vi "LabVIEW RTE Debugging Viewer.vi"() -> ()   [LabVIEW 2015]
panel:
  in  "use default":bool=TRUE
  in  "Application to Debug":u16(ring)
  in  "autoRefresh":bool=TRUE
  in  "Refresh Button":bool
  in  "VIs Currently Loaded in Selected Application":i32(listbox)
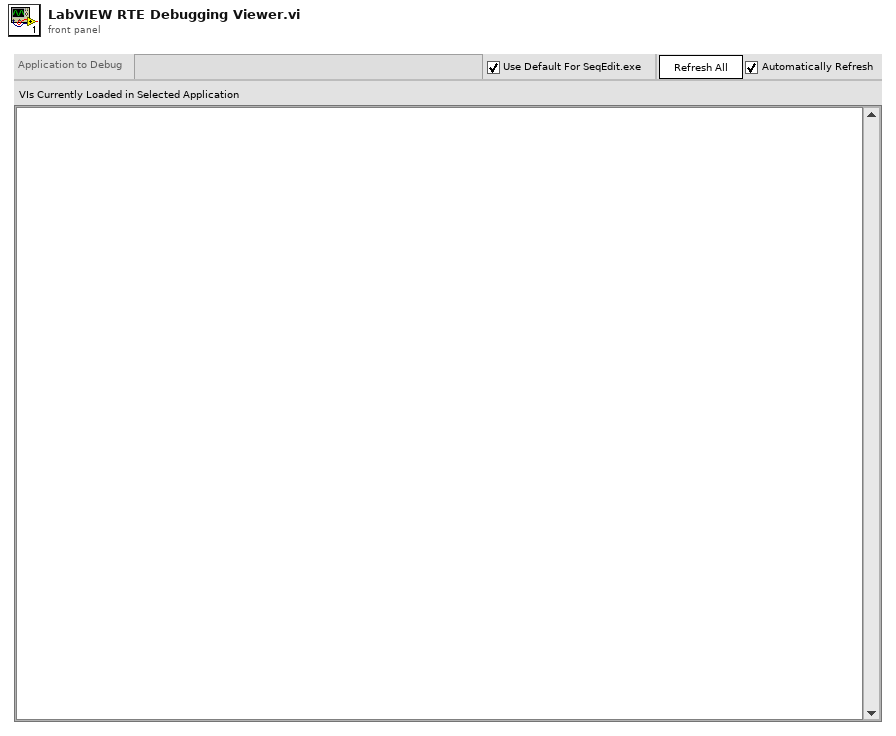
[diagram p1: front panel]
types:
  T1 = enum8{"Enabled", "Disabled", "Disabled and Grayed Out"}
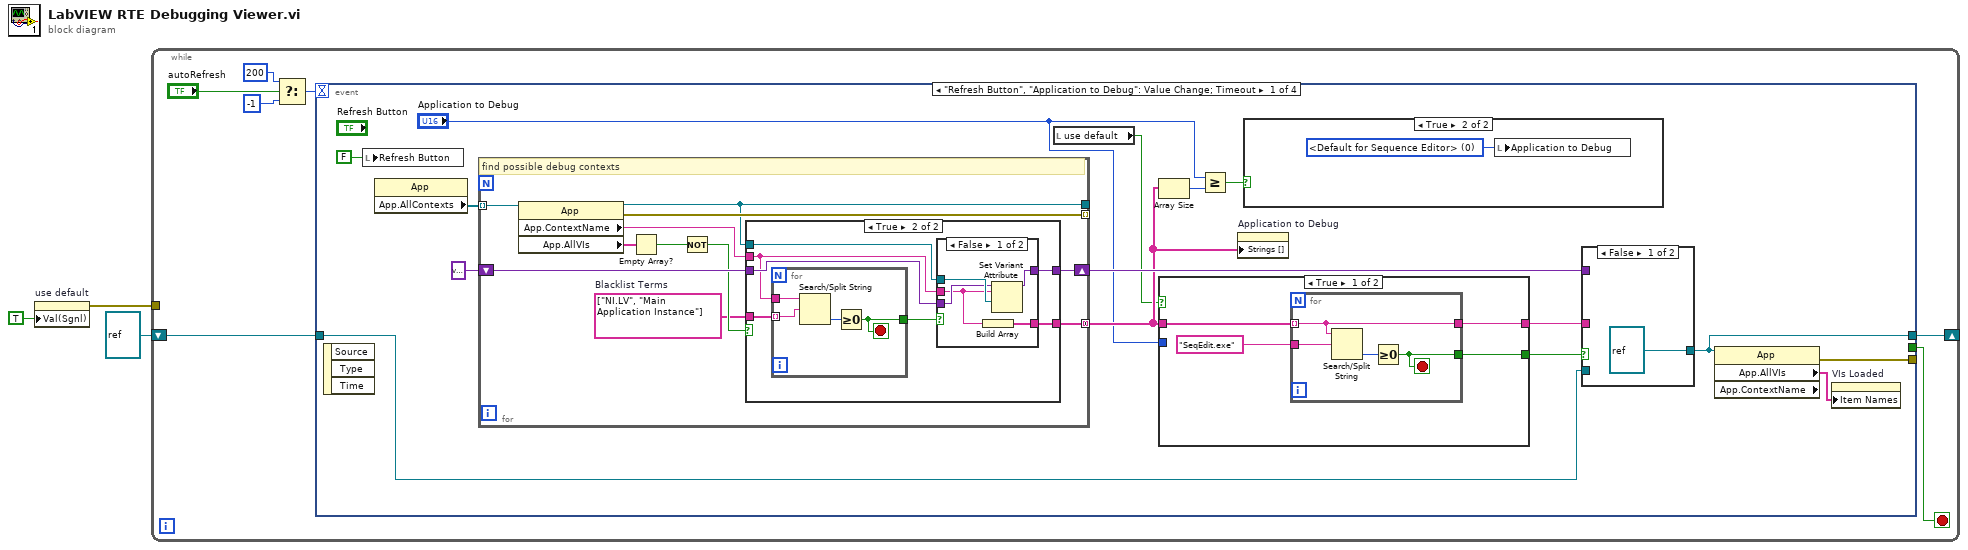
[diagram p0: block diagram]
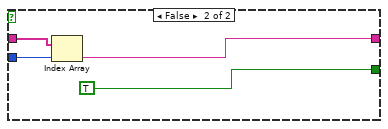
[diagram p5: hidden frame]
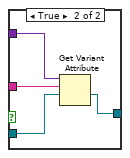
[diagram p6: hidden frame]
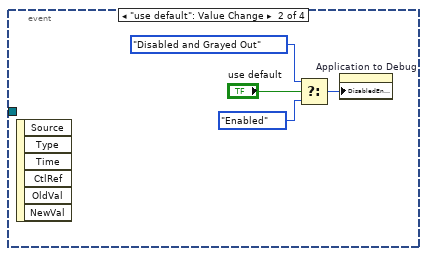
[diagram p7: hidden frame]
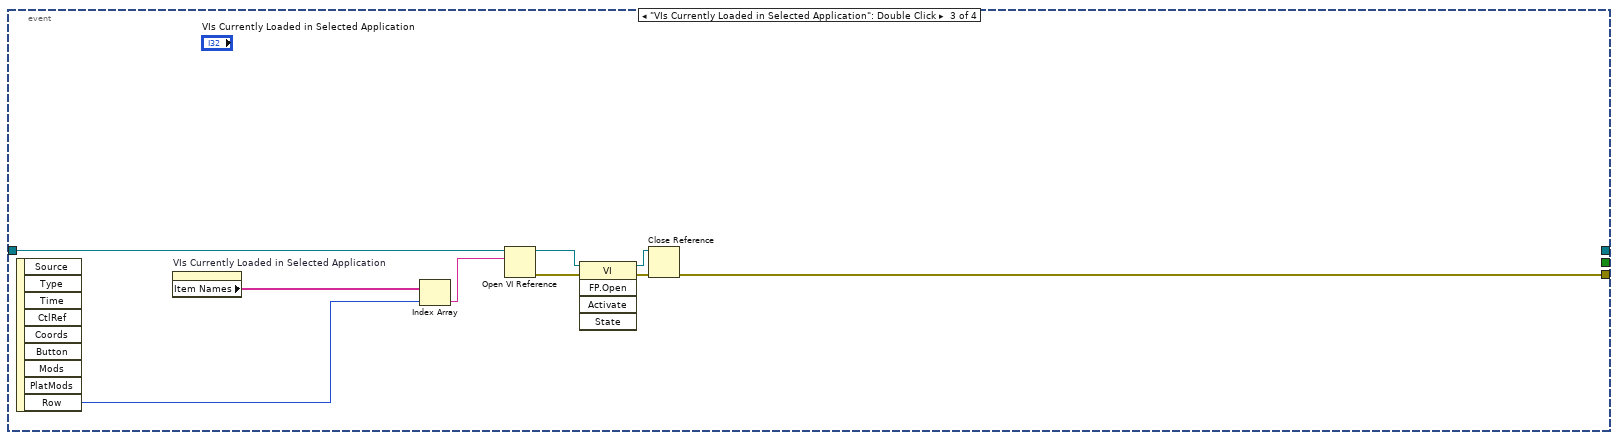
[diagram p8: hidden frame]
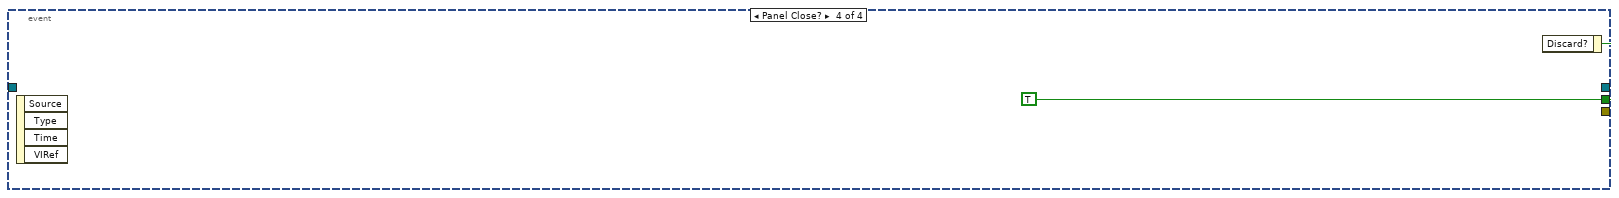
[diagram p9: hidden frame]
diagram:
  n1 = property on="use default" class="Bool (strict)"("Val(Sgnl)"=TRUE ("Value (Signaling)")) -> (error out=w1:errorcluster)  [unwired: 2 in, 1 out]
  n2 = while {
    shift-right: [w8] -> _
    shift-left: refnum<vi> refnum -> [w9]
    tunnel: w1 -> [_]
    stop <- w10 stop-if-true
    n3 = Select(t=200, s="autoRefresh", f=-1) -> (s? t:f=w4:i32)
    n4 = event shown="[0] \"Refresh Button\", \"Application to Debug\": Value Change;  Timeout" {
      selector: _ -> [_ _ _ _]
      dyn-events: _ -> [_ _ _ _]
      timeout: w4 -> [_ _ _ _]
      tunnel: [_ _ _ w86] -> w10
      tunnel: w9 -> [w17 _ w81 _]
      tunnel: [w16 _ _ _] -> w8
      tunnel: [w21 _ w77 _] -> _
      event "Refresh Button", "Application to Debug": Value Change; Timeout {
        n5 = event-data() -> ()  [unwired: 1 in, 3 out]
        n6 = local write "Refresh Button"(FALSE ("Refresh Button")) -> ()
        n7 = property class="App"() -> ("App.AllContexts"=w24:refnum<vi>[])  [unwired: 2 in, 2 out]
        n8 = for {
          tunnel: w24 -> [w36] mode=indexing
          tunnel: [w34] -> _
          tunnel: [w35] -> _ mode=indexing
          shift-right: [w32] -> w18
          shift-left: variant -> [w33]
          tunnel: [w27] -> w13 mode=concatenating
          w26 = string[] ["NI.LV", "Main Application Instance"]  # Blacklist Terms
          # "find possible debug contexts"
          n9 = property class="App"(reference=w36) -> (reference out=w34:refnum<vi>, error out=w35:errorcluster, "App.ContextName"=w31:string, "App.AllVIs"=w30:string[])  [unwired: 1 in]
          n10 = Empty Array?(array=w30) -> (empty?=w29:bool)
          n11 = Not(x=w29) -> (.not. x?=w28:bool)
          n12 = case shown="True" w28 {
            tunnel: w34 -> [_ w44]
            tunnel: w33 -> [w37 w43]
            tunnel: [w37 w42] -> w32
            tunnel: w31 -> [_ w39]
            tunnel: [_ w41] -> w27
            tunnel: w26 -> [_ w40]
            frame False {
            }
            frame True {
              n13 = for {
                tunnel: w40 -> [w53] mode=indexing
                tunnel: w39 -> [w54]
                tunnel: [w51] -> w38
                stop <- w51 stop-if-true
                n14 = Search/Split String(string=w54, search string/char (-)=w53) -> (offset of match=w52:i32)  [unwired: 1 in, 2 out]
                n15 = Greater Or Equal To 0?(x=w52) -> (x >= 0?=w51:bool)
              }
              n16 = case shown="False" w38 {
                tunnel: w44 -> [w49 _]
                tunnel: w43 -> [w48 w50]
                tunnel: [w47 w50] -> w42
                tunnel: [w46 _] -> w41
                tunnel: w39 -> [w45 _]
                frame False {
                  n17 = Build Array(w45) -> (w46:string[])
                  n18 = Set Variant Attribute(Variant=w48, name=w45, value=w49) -> (Variant out=w47:variant)  [unwired: 1 in, 2 out]
                }
                frame True {
                }
              }
            }
          }
        }
        n19 = local read "use default"() -> (w12:bool)
        n20 = Array Size(array=w13) -> (size(s)=w15:i32)
        n21 = case shown="True" w12 {
          tunnel: w13 -> [w57 w67]
          tunnel: [w59 w66] -> w20
          tunnel: [w58 TRUE] -> w19
          tunnel: "Application to Debug" -> [_ w64]
          frame True {
            n22 = for {
              tunnel: w57 -> [w62] mode=indexing
              tunnel: [w62] -> w59
              tunnel: "SeqEdit.exe" ("search string/char (-)") -> [w61]
              tunnel: [w60] -> w58
              stop <- w60 stop-if-true
              n23 = Search/Split String(string=w62, search string/char (-)=w61) -> (offset of match=w63:i32)  [unwired: 1 in, 2 out]
              n24 = Greater Or Equal To 0?(x=w63) -> (x >= 0?=w60:bool)
            }
          }
          frame False {
            n25 = Index Array(array=w67, index=w64) -> (element=w66:string)
          }
        }
        n26 = Greater Or Equal?(x="Application to Debug", y=w15) -> (x >= y?=w14:bool)
        n27 = property on="Application to Debug" class="Ring (strict)"("Strings []"=w13) -> ()  [unwired: 2 in, 2 out]
        n28 = case shown="True" w14 {
          frame False {
          }
          frame True {
            w55 = u16 0 items=["<Default for Sequence Editor>"] ("Application to Debug")
            n29 = local write "Application to Debug"(w55) -> ()
          }
        }
        n30 = case shown="False" w19 {
          tunnel: w18 -> [_ w72]
          tunnel: w17 -> [_ w71]
          tunnel: [refnum<vi> refnum w70] -> w16
          tunnel: w20 -> [_ w69]
          frame False {
          }
          frame True {
            n31 = Get Variant Attribute(Variant=w72, name=w69, default value (empty Variant)=w71) -> (value=w70:refnum<vi>)  [unwired: 1 in, 3 out]
          }
        }
        n32 = property class="App" props=["App.AllVIs", "App.ContextName"](reference=w16) -> (error out=w21:errorcluster, "App.AllVIs"=w25:string[])  [unwired: 1 in, 2 out]
        n33 = property on="VIs Loaded" class="LstBox (strict)"("Item Names"=w25) -> ()  [unwired: 2 in, 2 out]
      }
      event "use default": Value Change {
        n34 = event-data() -> ()  [unwired: 1 in, 6 out]
        n35 = Select(t=T1."Disabled and Grayed Out" ("Disabled"), s="use default", f=T1."Enabled" ("Disabled")) -> (s? t:f=w73:T1)
        n36 = property on="Application to Debug" class="Ring (strict)"("DisabledEnum"=w73) -> ()  [unwired: 2 in, 2 out]
      }
      event "VIs Currently Loaded in Selected Application": Double Click {
        n37 = event-data() -> ("Row"=w85:i32)  [unwired: 1 in, 8 out]
        n38 = property on="VIs Currently Loaded in Selected Application" class="LstBox (strict)"() -> ("Item Names"=w84:string[])  [unwired: 2 in, 2 out]
        n39 = Index Array(array=w84, index=w85) -> (element=w83:string)
        n40 = Open VI Reference(application reference (local)=w81, vi path=w83) -> (vi reference=w82:refnum<vi>, error out=w80:errorcluster)  [unwired: 4 in]
        n41 = invoke class="VI" method="FP.Open"(reference=w82, error in=w80) -> (reference out=w78:refnum<vi>, error out=w79:errorcluster)  [unwired: 3 in, 3 out]
        n42 = Close Reference(reference=w78, error in (no error)=w79) -> (error out=w77:errorcluster)
      }
      event Panel Close? {
        w86 = TRUE ("Discard?")
        n43 = event-data() -> ()  [unwired: 1 in, 4 out]
        n44 = event-data("Discard?"=w86) -> ()  [unwired: 1 in, 1 out]
      }
    }
  }
